vi "SpinnyCurrentPos.vi"(0 "Arduino Resource":T1={"VISA resource"="", "Board Type"=enum."Uno", "Connection Type"=enum."USB / Serial", "Bytes Per Packet (15)"=15}, 3 "stepper #":u8=1, 5 "error in":errorcluster) -> (14 "Arduino Resource Out":T1={"VISA resource"="", "Board Type"=enum."Uno", "Connection Type"=enum."USB / Serial", "Bytes Per Packet (15)"=15}, 18 "position":i32, 19 "error out":errorcluster)   [LabVIEW 2014]
doc: "return current position of nth stepper in steps"
uses:
  <vilib>/LabVIEW Interface for Arduino/Type Defs/Arduino Resource.ctl
  <vilib>/LabVIEW Interface for Arduino/Type Defs/Board Type.ctl
  <vilib>/LabVIEW Interface for Arduino/LabVIEW Interface for Arduino.lvlib
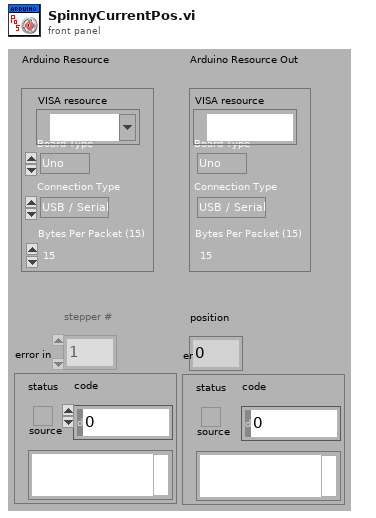
[diagram p1: front panel]
types:
  T1 = typedef "LabVIEW Interface for Arduino.lvlib/Arduino Resource.ctl" = cluster{"VISA resource":refnum<visa-resource-name>, "Board Type":T2, "Connection Type":enum8{"USB / Serial"}, "Bytes Per Packet (15)":u8}
  T2 = typedef "LabVIEW Interface for Arduino.lvlib/Board Type.ctl" = enum16{"Uno", "Dimuelanove w/Atmega 328", "Mega 2560"}
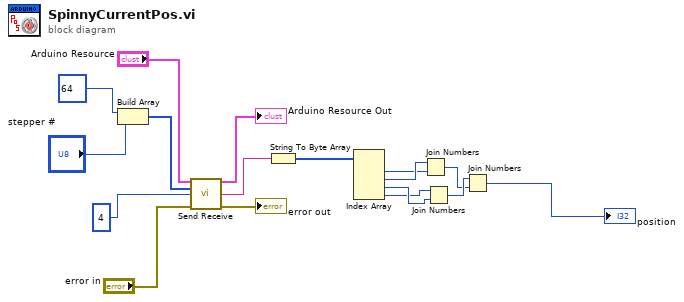
[diagram p0: block diagram]
diagram:
  n1 = Build Array(u8 64, "stepper #") -> (w11:u8[])
  n2 = call <vilib>:"Send Receive.vi"("Arduino Resource"="Arduino Resource", "Data"=w11, "Bytes To Read (0)"=u8 4, "error in"="error in") -> ("Arduino Resource"=→"Arduino Resource Out":T1, "Read Buffer"=w10:string, "error out"=→"error out":errorcluster)  [unwired: 9 in]
  n3 = String To Byte Array(string=w10) -> (unsigned byte array=w9:u8[])
  n4 = Index Array(array=w9) -> (element #1=w7:u8, element #2=w8:u8, element #3=w5:u8, element #4=w4:u8)  [unwired: 4 in]
  n5 = Join Numbers(hi=w8, lo=w7) -> ((hi.lo)=w2:u16)
  n6 = Join Numbers(hi=w4, lo=w5) -> ((hi.lo)=w3:u16)
  n7 = Join Numbers(hi=w3, lo=w2) -> ((hi.lo)=→"position":u32)
